vi "ACNET Monitor.vi"() -> ()   [LabVIEW 2013]
uses:
  ACNET Monitor/ACNET Devices.lvclass
  user.lib/Merge Sort String Arrays.vi
  ACNET Monitor.lvlib
  <vilib>/httpClient/LabVIEWHTTPClient.lvlib
panel:
  out "State Changed":bool
  in  "stop":bool
  out "Updating":bool
  in  "Tab Control":T1(tab)
  in  "Available Devices":i32[](listbox)
  in  "Remove from Monitor List":bool
  in  "Monitor":bool
  in  "Monitoring":i32[](listbox)
  out "description":string
  out "min value":dbl
  out "max value":dbl
  out "current value":dbl
  out "name":string
  out "units":string
  in  "Summary":i32[](listbox)
  in  "Update Period (seconds)":u32=5
  in  "Configuration File":path=path "C:/Users/plane/Dropbox/Research/MTA/DAQ VIs/MTA Shift Toolbox/device_limits_personal.xml"
  in  "Out-of-range State File":path=path "C:/Users/plane/Desktop/ACNET/acnet_monitor_state.txt"
  in  "Out-of-Range Alert Sound File":path=path "C:/Users/plane/Dropbox/Research/MTA/DAQ VIs/MTA Shift Toolbox/alertklaxon_clean.wav"
  in  "Back-in-Range Alert Sound File":path=path "C:/Users/plane/Dropbox/Research/MTA/DAQ VIs/MTA Shift Toolbox/tng-data-allsystems.wav"
  in  "Notification Email Recipients":string[](array[string])
  out "ACNET Error":errorcluster
  out "Monitored Devices":refnum<class "ACNET Devices.lvclass">
  out "Range Check Results":T2(array[cluster])
  out "Devices":refnum<class "ACNET Devices.lvclass">
  # "ACNET Monitor.vi\nupdated on 5 Apr 2015\nby P. Lane"
  # "TODO:\nx 1) Play alarm sound if there are any out-of-range devices\nx 2) Email shifter (initially just have a textbox control)\n3) Add shifter database support for email notifications"
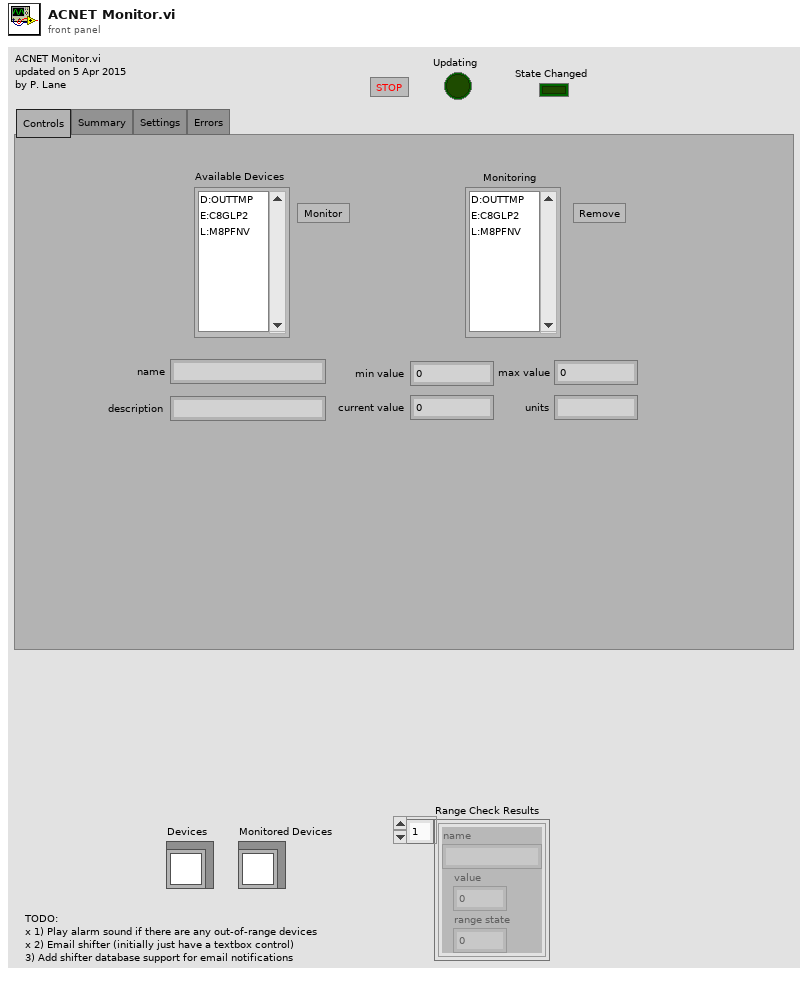
[diagram p1: front panel]
types:
  T1 = enum32{"Controls", "Summary", "Settings", "Errors"}
  T2 = cluster{"name":string, "value":dbl, "range state":i8}[]
  T3 = enum16{"open", "replace", "create", "open or create", "replace or create", "replace or create with confirmation"}
  T4 = typedef "LabVIEWHTTPClient.lvlib/ClientHandle.ctl" = refnum<k1>
  T5 = cluster{"Devices":refnum<vi>, "Range Check Results":refnum<vi>, "Listbox":refnum<vi>}
  T6 = cluster{"name":refnum<vi>, "description":refnum<vi>, "min value":refnum<vi>, "max value":refnum<vi>, "current value":refnum<vi>, "units":refnum<vi>}
  T7 = cluster{"name":string, "value":dbl, "range state":i8}
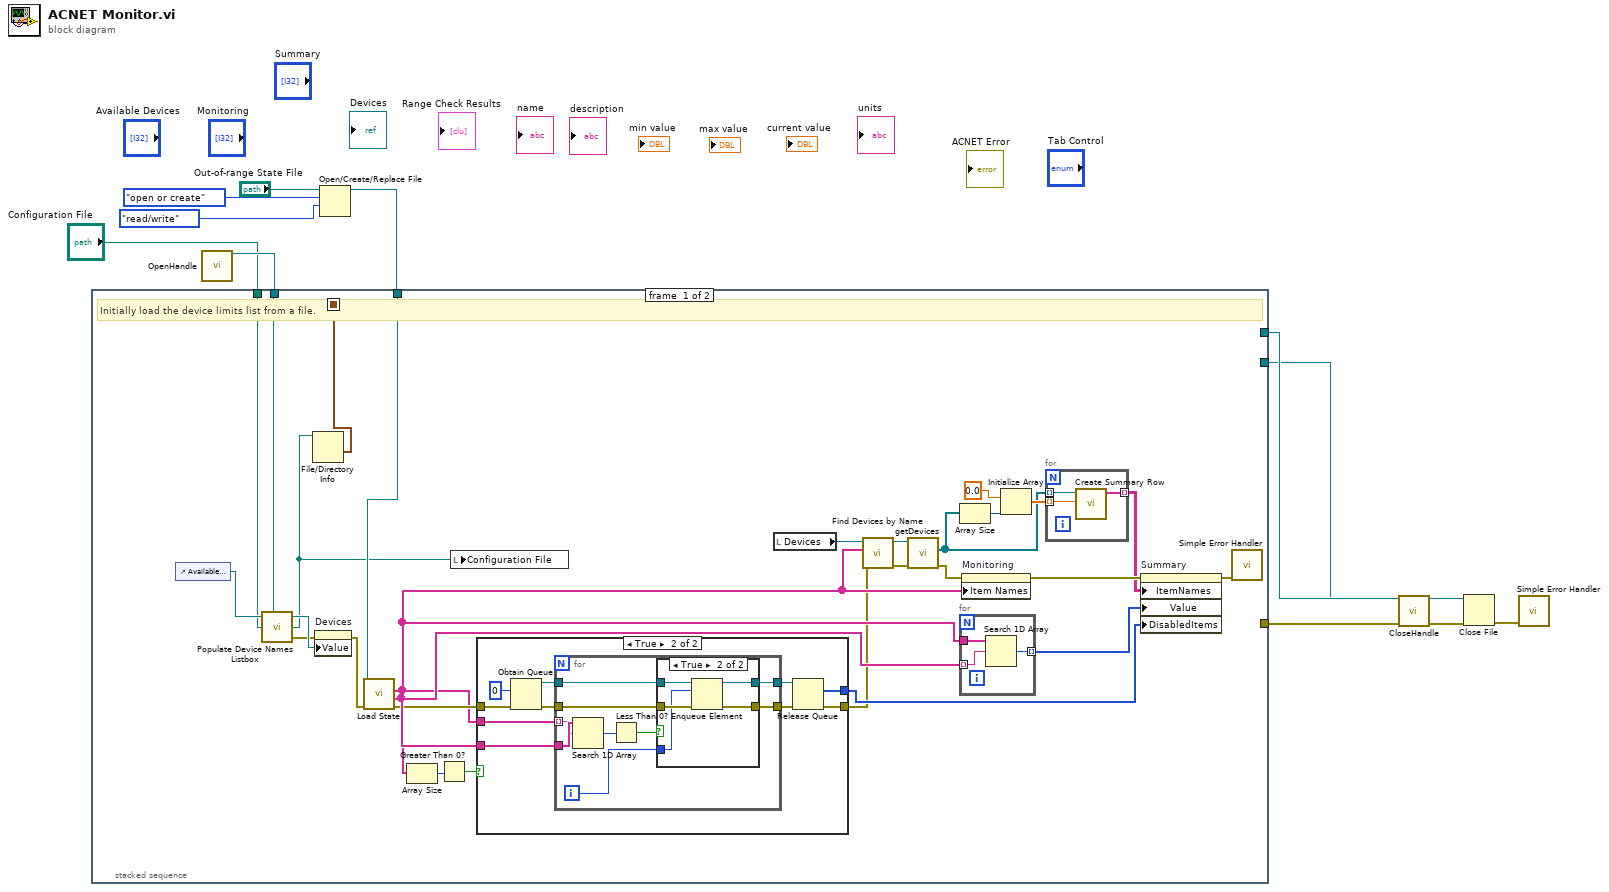
[diagram p0: block diagram]
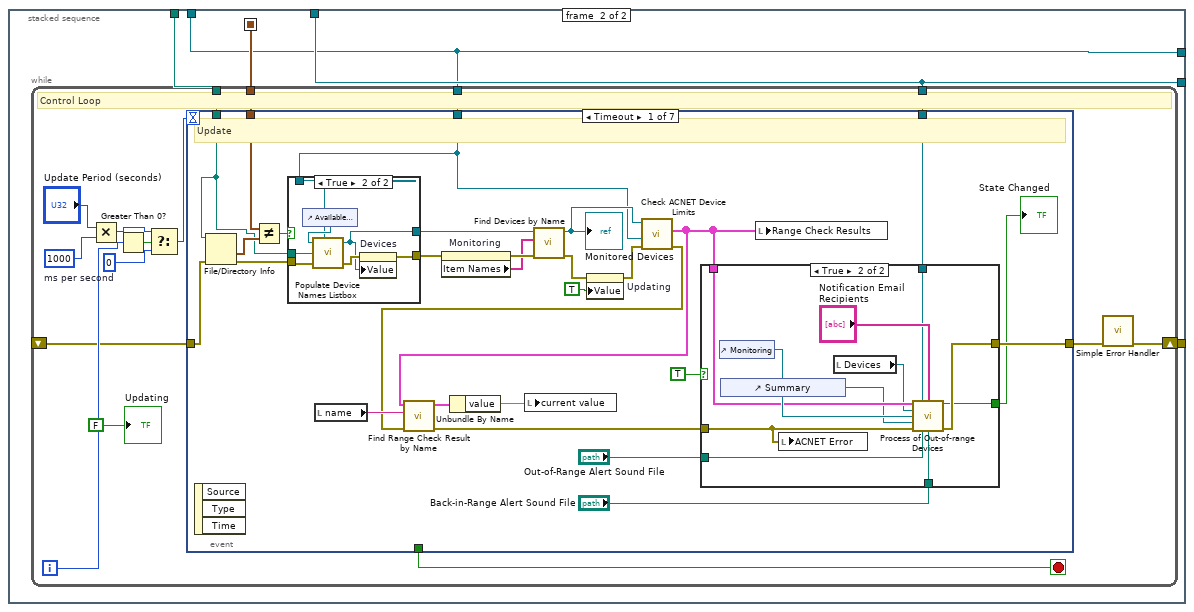
[diagram p4: hidden frame]
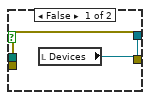
[diagram p5: hidden frame]
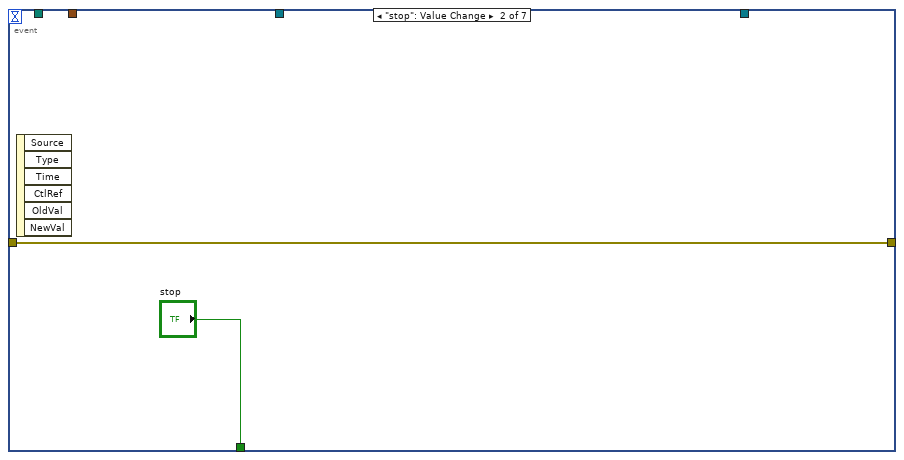
[diagram p7: hidden frame]
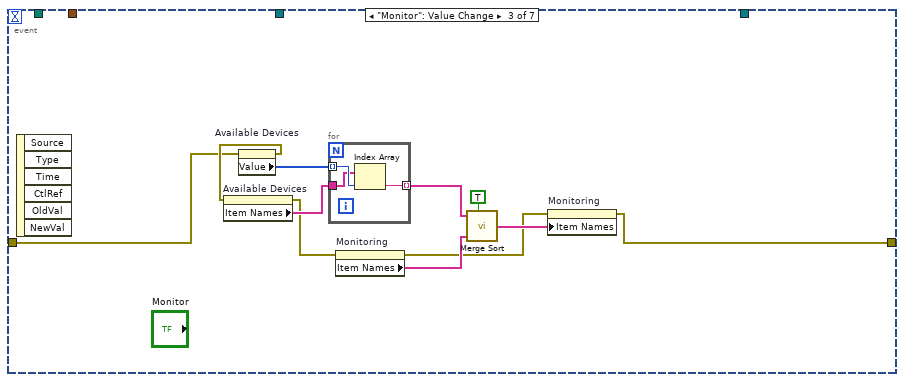
[diagram p8: hidden frame]
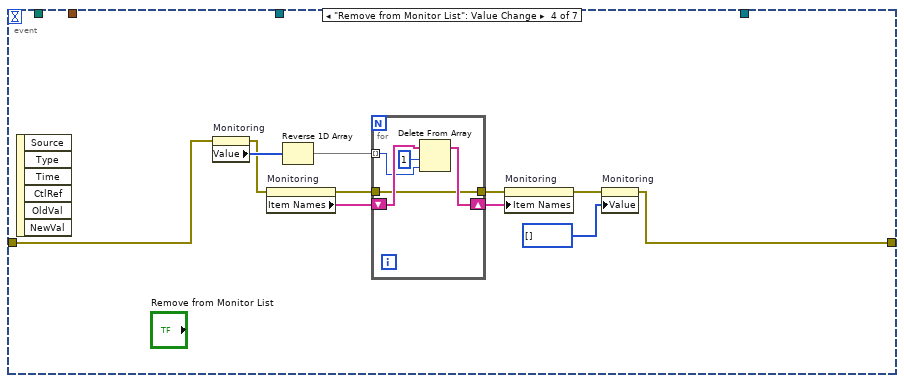
[diagram p9: hidden frame]
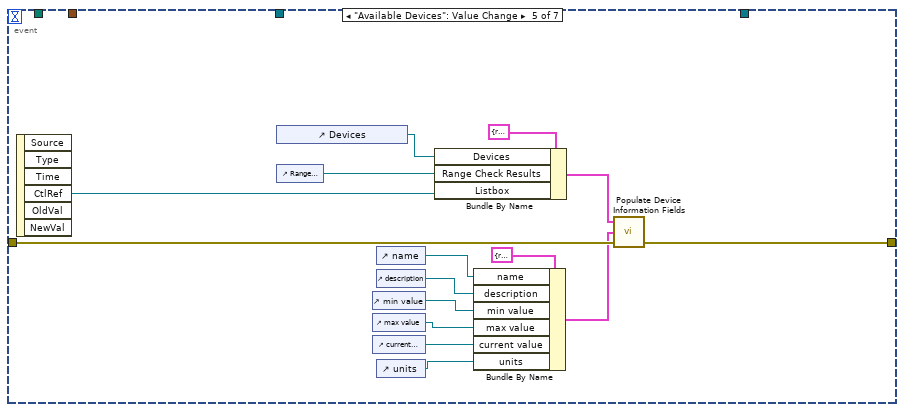
[diagram p10: hidden frame]
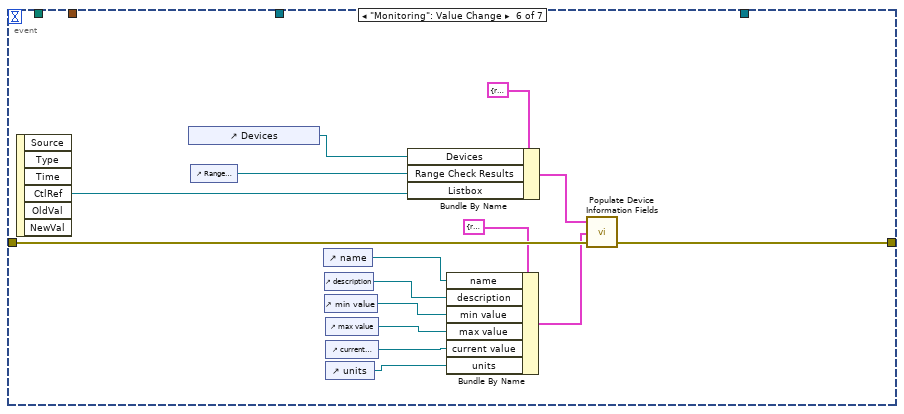
[diagram p11: hidden frame]
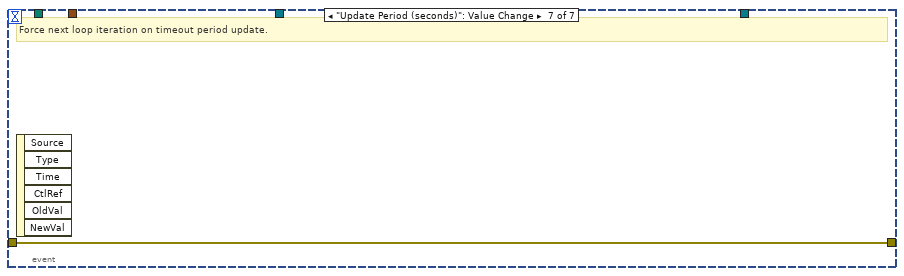
[diagram p12: hidden frame]
diagram:
  n1 = call <vilib>:"OpenHandle.vi"() -> ("client handle out"=w2:T4)  [unwired: 14 in, 1 out]
  n2 = Open/Create/Replace File(file path (use dialog)="Out-of-range State File", operation (0:open)=T3."open or create", access (0:read/write)=enum16{"read/write", "read-only", "write-only"}."read/write") -> (refnum out=w3:refnum<file>)  [unwired: 3 in, 2 out]
  n3 = stacked-sequence {
    seq-local: [w30 _] -> [_ w75]
    tunnel: [_ w76] -> w10
    tunnel: [_ w73] -> w11
    tunnel: [_ w74] -> w9
    tunnel: w3 -> [w28 w74]
    tunnel: w2 -> [w26 w73]
    tunnel: "Configuration File" -> [w23 w72]
    frame #0 {
      # "Initially load the device limits list from a file."
      n4 = control-ref of="Available Devices"() -> (w38:refnum<vi>)
      n5 = call "Populate Device Names Listbox.vi"("LstBox Refnum"=w38, "client handle"=w26, "XML File Path"=w23) -> ("ACNET Devices out"=w33:refnum<class "ACNET Devices.lvclass">, "XML File Path (duplicate)"=w24:path, "error out"=w27:errorcluster)  [unwired: 2 in]
      n6 = File/Directory Info(path=w24) -> (last mod=w30:timestamp)  [unwired: 1 in, 6 out]
      n7 = property on="Devices" class="LVClassControl (strict)"(error in=w27, "Value"=w33) -> ()  [unwired: 1 in, 2 out]
      n8 = call "Load State.vi"("error in"=w27, "State File Refnum"=w28) -> ("error out"=w29:errorcluster, "Out-of-range List"=w35:string[], "Monitoring List"=w16:string[])  [unwired: 6 in, 1 out]
      n9 = Array Size(array=w16) -> (size(s)=w32:i32)
      n10 = Greater Than 0?(x=w32) -> (x > 0?=w31:bool)
      n11 = local write "Configuration File"(w24) -> ()
      n12 = case shown="True" w31 {
        tunnel: w16 -> [_ w49]
        tunnel: w35 -> [_ w48]
        tunnel: [_ w45] -> w34
        tunnel: w29 -> [w42 w44]
        tunnel: [w42 w43] -> w15
        frame False {
        }
        frame True {
          n13 = Obtain Queue(element data type=0 ("index of element"), error in (no error)=w44) -> (queue out=w51:refnum<queue>, error out=w50:errorcluster)  [unwired: 3 in, 1 out]
          n14 = for {
            tunnel: w51 -> [w60]
            tunnel: w50 -> [w61]
            tunnel: [w59] -> w46
            tunnel: [w58] -> w47
            tunnel: w49 -> [w56] mode=indexing
            tunnel: w48 -> [w57]
            i -> [w53]
            n15 = Search 1D Array(1D array=w57, element=w56) -> (index of element=w55:i32)  [unwired: 1 in]
            n16 = Less Than 0?(x=w55) -> (x < 0?=w54:bool)
            n17 = case shown="True" w54 {
              tunnel: w61 -> [w63 w68]
              tunnel: w60 -> [w62 w67]
              tunnel: [w62 w66] -> w59
              tunnel: [w63 w65] -> w58
              tunnel: w53 -> [_ w64]
              frame False {
              }
              frame True {
                n18 = Enqueue Element(queue=w67, element=w64, error in (no error)=w68) -> (queue out=w66:refnum<queue>, error out=w65:errorcluster)  [unwired: 1 in, 1 out]
              }
            }
          }
          n19 = Release Queue(queue=w46, error in (no error)=w47) -> (remaining elements=w45:i32[], error out=w43:errorcluster)  [unwired: 1 in, 1 out]
        }
      }
      n20 = local read "Devices"() -> (w17:refnum<class "ACNET Devices.lvclass">)
      n21 = call "Find Devices by Name.vi"("error in"=w15, "Device Names"=w16, "ACNET Devices in"=w17) -> ("error out"=w19:errorcluster, "ACNET Devices out"=w18:refnum<class "ACNET Devices.lvclass">)  [unwired: 7 in]
      n22 = call-dynamic "getDevices.vi"("error in (no error)"=w19, "ACNET Devices in"=w18) -> ("error out"=w14:errorcluster, "Devices"=w13:refnum<class "ACNET Device.lvclass">[])  [unwired: 7 in, 1 out]
      n23 = Array Size(array=w13) -> (size(s)=w22:i32)
      n24 = for {
        tunnel: w35 -> [w71] mode=indexing
        tunnel: w16 -> [w70]
        tunnel: [w69] -> w36 mode=indexing
        n25 = Search 1D Array(1D array=w70, element=w71) -> (index of element=w69:i32)  [unwired: 1 in]
      }
      n26 = property on="Monitoring" class="LstBox (strict)"(error in=w14, "Item Names"=w16) -> (error out=w37:errorcluster)  [unwired: 1 in, 1 out]
      n27 = Initialize Array(0.0 ("value"), w22) -> (w20:dbl[])
      n28 = for {
        tunnel: w13 -> [w41] mode=indexing
        tunnel: w20 -> [w40] mode=indexing
        tunnel: [w39] -> w12 mode=indexing
        n29 = call "Create Summary Row.vi"("value"=w40, "ACNET Device.lvclass"=w41) -> ("Summary Row"=w39:string[])  [unwired: 8 in, 1 out]
      }
      n30 = property on="Summary" class="MCListbox (strict)"(error in=w37, "ItemNames"=w12, "Value"=w36, "DisabledItems"=w34) -> (error out=w25:errorcluster)  [unwired: 1 in, 1 out]
      n31 = call <vilib>:"Simple Error Handler.vi"("error in (no error)"=w25) -> ()  [unwired: 4 in, 5 out]
    }
    frame #1 {
      n32 = while {
        shift-right: [w77] -> w76
        shift-left: _ -> [w79]
        tunnel: w73 -> [w83]
        tunnel: w72 -> [w82]
        tunnel: w75 -> [w81]
        tunnel: w74 -> [w80]
        i -> [w88]
        stop <- w92 stop-if-true
        w91 = u32 1000  # ms per second
        # "Control Loop"
        n33 = Multiply(x="Update Period (seconds)", y=w91) -> (x*y=w86:u32)
        n34 = Greater Than 0?(x=w88) -> (x > 0?=w87:bool)
        n35 = Select(t=w86, s=w87, f=u32 0) -> (s? t:f=w84:u32)
        n36 = event shown="[0] Timeout" {
          selector: _ -> [_ _ _ _ _ _ _]
          dyn-events: _ -> [_ _ _ _ _ _ _]
          timeout: w84 -> [_ _ _ _ _ _ _]
          tunnel: [_ "stop" _ _ _ _ _] -> w92
          tunnel: w79 -> [w106 w141 w143 w158 w184 w198 w203]
          tunnel: [w118 w141 w144 w157 w175 w193 w203] -> w78
          tunnel: w83 -> [w93 _ _ _ _ _ _]
          tunnel: w82 -> [w109 _ _ _ _ _ _]
          tunnel: w81 -> [w111 _ _ _ _ _ _]
          tunnel: w80 -> [w107 _ _ _ _ _ _]
          event Timeout {
            # "Update"
            n37 = event-data() -> ()  [unwired: 1 in, 3 out]
            n38 = File/Directory Info(path=w109, error in=w106) -> (last mod=w112:timestamp, error out=w108:errorcluster)  [unwired: 5 out]
            n39 = Not Equal?(x=w111, y=w112) -> (x != y?=w110:bool)
            n40 = case shown="True" w110 {
              tunnel: w109 -> [_ w128]
              tunnel: [w121 w126] -> w103
              tunnel: w108 -> [w120 w125]
              tunnel: [w120 w124] -> w105
              tunnel: w93 -> [_ w122]
              frame False {
                n41 = local read "Devices"() -> (w121:refnum<class "ACNET Devices.lvclass">)
              }
              frame True {
                n42 = control-ref of="Available Devices"() -> (w123:refnum<vi>)
                n43 = call "Populate Device Names Listbox.vi"("LstBox Refnum"=w123, "client handle"=w122, "XML File Path"=w128, "error in (no error)"=w125) -> ("ACNET Devices out"=w126:refnum<class "ACNET Devices.lvclass">, "error out"=w127:errorcluster)  [unwired: 1 in, 1 out]
                n44 = property on="Devices" class="LVClassControl (strict)"(error in=w127, "Value"=w126) -> (error out=w124:errorcluster)  [unwired: 1 in, 1 out]
              }
            }
            n45 = local read "name"() -> (w99:string)
            n46 = property on="Monitoring" class="LstBox (strict)"(error in=w105) -> (error out=w104:errorcluster, "Item Names"=w102:string[])  [unwired: 1 in, 1 out]
            n47 = call "Find Devices by Name.vi"("error in"=w104, "Device Names"=w102, "ACNET Devices in"=w103) -> ("error out"=w100:errorcluster, "ACNET Devices out"=w101:refnum<class "ACNET Devices.lvclass">)  [unwired: 7 in]
            "Monitored Devices" <- w101
            n48 = property on="Updating" class="Bool (strict)"(error in=w100, "Value"=TRUE ("Updating")) -> (error out=w113:errorcluster)  [unwired: 1 in, 1 out]
            n49 = call "Check ACNET Device Limits.vi"("error in (no error)"=w113, "client handle"=w93, "ACNET Devices in"=w101) -> ("error out"=w98:errorcluster, "Range Check Results"=w96:T2)  [unwired: 5 in, 2 out]
            n50 = call "Find Range Check Result by Name.vi"("error in"=w98, "Device Name"=w99, "Range Check Results in"=w96) -> ("error out"=w97:errorcluster, "Range Check Result out"=w95:T7)  [unwired: 6 in, 1 out]
            n51 = Unbundle By Name(w95) -> ("value"=w94:dbl)
            n52 = local write "current value"(w94) -> ()
            n53 = case shown="True" TRUE {
              tunnel: [w129 w140] -> w118
              tunnel: w97 -> [w129 w133]
              tunnel: "Out-of-Range Alert Sound File" -> [_ w138]
              tunnel: [_ w137] -> w116
              tunnel: "Back-in-Range Alert Sound File" -> [_ w136]
              tunnel: w96 -> [_ w134]
              tunnel: w107 -> [_ w132]
              frame False {
              }
              frame True {
                n54 = control-ref of="Monitoring"() -> (w139:refnum<vi>)
                n55 = control-ref of="Summary"() -> (w131:refnum<vi>)
                n56 = local write "ACNET Error"(w133) -> ()
                n57 = local read "Devices"() -> (w130:refnum<class "ACNET Devices.lvclass">)
                n58 = call "Process of Out-of-range Devices.vi"("Range Check Results"=w134, "State File Refnum"=w132, "Recipients"="Notification Email Recipients", "Devices"=w130, "Monitoring Listbox"=w139, "Summary Listbox"=w131, "error in (no error)"=w133, "Out-of-Range Alert Sound File"=w138, "Back-in-Range Alert Sound File"=w136) -> ("State Changed"=w137:bool, "error out"=w140:errorcluster)  [unwired: 5 in]
              }
            }
            "State Changed" <- w116
            n59 = local write "Range Check Results"(w96) -> ()
          }
          event "stop": Value Change {
            n60 = event-data() -> ()  [unwired: 1 in, 6 out]
          }
          event "Monitor": Value Change {
            n61 = event-data() -> ()  [unwired: 1 in, 6 out]
            n62 = property on="Available Devices" class="LstBox (strict)"(error in=w143) -> (error out=w148:errorcluster, "Value"=w153:i32[])  [unwired: 1 in, 1 out]
            n63 = property on="Available Devices" class="LstBox (strict)"(error in=w148) -> (error out=w147:errorcluster, "Item Names"=w152:string[])  [unwired: 1 in, 1 out]
            n64 = for {
              tunnel: w153 -> [w156] mode=indexing
              tunnel: w152 -> [w155]
              tunnel: [w154] -> w151 mode=indexing
              n65 = Index Array(array=w155, index=w156) -> (element=w154:string)
            }
            n66 = property on="Monitoring" class="LstBox (strict)"(error in=w147) -> (error out=w146:errorcluster, "Item Names"=w150:string[])  [unwired: 1 in, 1 out]
            n67 = call-poly "Merge Sort.vi"("String Array A"=w151, "Ignore Duplicates? (F)"=TRUE, "String Array B"=w150) -> ("Sorted String Array"=w149:string[])  [unwired: 4 in]
            n68 = property on="Monitoring" class="LstBox (strict)"(error in=w146, "Item Names"=w149) -> (error out=w144:errorcluster)  [unwired: 1 in, 1 out]
          }
          event "Remove from Monitor List": Value Change {
            n69 = event-data() -> ()  [unwired: 1 in, 6 out]
            n70 = property on="Monitoring" class="LstBox (strict)"(error in=w158) -> (error out=w163:errorcluster, "Value"=w167:i32[])  [unwired: 1 in, 1 out]
            n71 = property on="Monitoring" class="LstBox (strict)"(error in=w163) -> (error out=w162:errorcluster, "Item Names"=w165:string[])  [unwired: 1 in, 1 out]
            n72 = Reverse 1D Array(array=w167) -> (reversed array=w166:i32[])
            n73 = for {
              tunnel: w166 -> [w170] mode=indexing
              shift-right: [w169] -> w164
              shift-left: w165 -> [w171]
              tunnel: w162 -> [w168]
              tunnel: [w168] -> w161
              n74 = Delete From Array(array=w171, length=1, index=w170) -> (array with subset deleted=w169:string[])  [unwired: 1 out]
            }
            n75 = property on="Monitoring" class="LstBox (strict)"(error in=w161, "Item Names"=w164) -> (error out=w160:errorcluster)  [unwired: 1 in, 1 out]
            n76 = property on="Monitoring" class="LstBox (strict)"(error in=w160, "Value"=i32[] [] ("Monitor List")) -> (error out=w157:errorcluster)  [unwired: 1 in, 1 out]
          }
          event "Available Devices": Value Change {
            n77 = event-data() -> ("CtlRef"=w186:refnum<vi>)  [unwired: 1 in, 5 out]
            n78 = control-ref of="Devices"() -> (w173:refnum<vi>)
            n79 = control-ref of="Range Check Results"() -> (w185:refnum<vi>)
            n80 = control-ref of="min value"() -> (w181:refnum<vi>)
            n81 = control-ref of="max value"() -> (w180:refnum<vi>)
            n82 = control-ref of="current value"() -> (w179:refnum<vi>)
            n83 = control-ref of="name"() -> (w183:refnum<vi>)
            n84 = control-ref of="description"() -> (w182:refnum<vi>)
            n85 = control-ref of="units"() -> (w176:refnum<vi>)
            n86 = Bundle By Name(cluster=T5 {"Devices"=refnum, "Range Check Results"=refnum, "Listbox"=refnum} ("Inputs"), "Devices"=w173, "Range Check Results"=w185, "Listbox"=w186) -> (w174:T5)
            n87 = Bundle By Name(cluster=T6 {"name"=refnum, "description"=refnum, "min value"=refnum, "max value"=refnum, "current value"=refnum, "units"=refnum} ("Outputs"), "name"=w183, "description"=w182, "min value"=w181, "max value"=w180, "current value"=w179, "units"=w176) -> (w178:T6)
            n88 = call "Populate Device Information Fields.vi"("error in (no error)"=w184, "Outputs"=w178, "Inputs"=w174) -> ("error out"=w175:errorcluster)  [unwired: 2 in]
          }
          event "Monitoring": Value Change {
            n89 = event-data() -> ("CtlRef"=w200:refnum<vi>)  [unwired: 1 in, 5 out]
            n90 = control-ref of="Devices"() -> (w199:refnum<vi>)
            n91 = control-ref of="Range Check Results"() -> (w197:refnum<vi>)
            n92 = control-ref of="name"() -> (w189:refnum<vi>)
            n93 = control-ref of="description"() -> (w188:refnum<vi>)
            n94 = control-ref of="min value"() -> (w196:refnum<vi>)
            n95 = control-ref of="max value"() -> (w195:refnum<vi>)
            n96 = control-ref of="current value"() -> (w194:refnum<vi>)
            n97 = control-ref of="units"() -> (w190:refnum<vi>)
            n98 = Bundle By Name(cluster=T5 {"Devices"=refnum, "Range Check Results"=refnum, "Listbox"=refnum} ("Inputs"), "Devices"=w199, "Range Check Results"=w197, "Listbox"=w200) -> (w201:T5)
            n99 = Bundle By Name(cluster=T6 {"name"=refnum, "description"=refnum, "min value"=refnum, "max value"=refnum, "current value"=refnum, "units"=refnum} ("Outputs"), "name"=w189, "description"=w188, "min value"=w196, "max value"=w195, "current value"=w194, "units"=w190) -> (w192:T6)
            n100 = call "Populate Device Information Fields.vi"("error in (no error)"=w198, "Outputs"=w192, "Inputs"=w201) -> ("error out"=w193:errorcluster)  [unwired: 2 in]
          }
          event "Update Period (seconds)": Value Change {
            # "Force next loop iteration on timeout period update."
            n101 = event-data() -> ()  [unwired: 1 in, 6 out]
          }
        }
        n102 = call <vilib>:"Simple Error Handler.vi"("error in (no error)"=w78) -> ("error out"=w77:errorcluster)  [unwired: 4 in, 4 out]
        "Updating" <- FALSE ("Updating")
      }
    }
  }
  n103 = call <vilib>:"CloseHandle.vi"("client handle"=w11, "error in (no error)"=w10) -> ("error out"=w8:errorcluster)  [unwired: 13 in]
  n104 = Close File(refnum=w9, error in=w8) -> (error out=w7:errorcluster)  [unwired: 1 out]
  n105 = call <vilib>:"Simple Error Handler.vi"("error in (no error)"=w7) -> ()  [unwired: 4 in, 5 out]
